vi "get results and parameters refs.vi"(8 "error in":errorcluster, 11 "VI in":refnum<vi>) -> (0 "error out":errorcluster, 2 "Results from processing ref out":refnum<vi>, 3 "Parameters to process ref out":refnum<vi>)   [LabVIEW 2013]
uses:
  <vilib>/Utility/traverseref.llb/TRef TravTarget.ctl
  <vilib>/Utility/traverseref.llb/VI Scripting - Traverse.lvlib
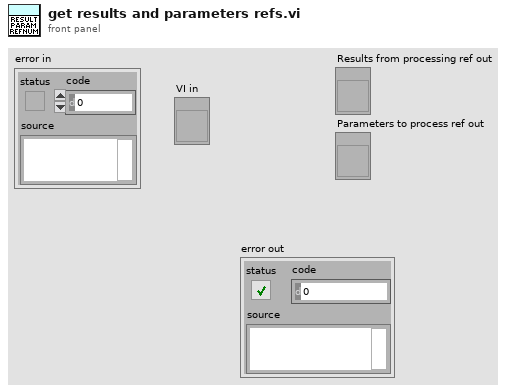
[diagram p1: front panel]
types:
  T1 = typedef "TRef TravTarget.ctl" = enum16{"FP", "BD", "Other"}
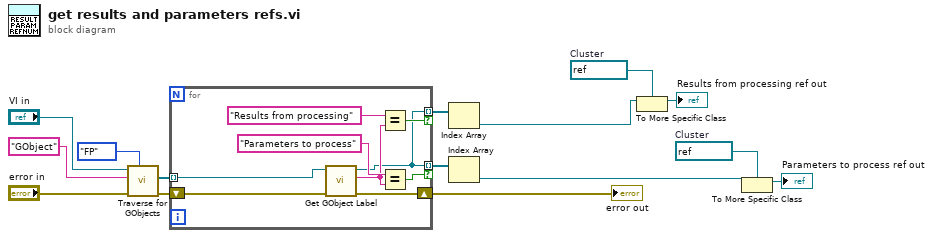
[diagram p0: block diagram]
diagram:
  w4 = refnum<vi> refnum  # Cluster
  w5 = refnum<vi> refnum  # Cluster
  n1 = call <vilib>:"Traverse for GObjects.vi"("Traverse Target"=TRef_TravTarget."FP", "error in (no error)"="error in", "Class Name"="GObject", "VI Refnum"="VI in") -> ("error out"=w14:errorcluster, "References"=w10:refnum<vi>[])  [unwired: 4 in, 2 out]
  n2 = for {
    tunnel: [w18] -> w12 mode=indexing if=w22
    shift-right: [w21] -> w13
    shift-left: w14 -> [w24]
    tunnel: [w18] -> w11 mode=indexing if=w17
    tunnel: w10 -> [w16] mode=indexing
    n3 = call <vilib>:"Get GObject Label.vi"("error in (no error)"=w24, "GObject"=w16) -> ("error out"=w21:errorcluster, "Object Label"=w19:string, "dup GObject"=w18:refnum<vi>)  [unwired: 5 in, 2 out]
    n4 = Equal?(x="Results from processing", y=w19) -> (x = y?=w22:bool)
    n5 = Equal?(x="Parameters to process", y=w19) -> (x = y?=w17:bool)
  }
  "error out" <- w13
  n6 = Index Array(array=w12) -> (element=w6:refnum<vi>)  [unwired: 1 in]
  n7 = Index Array(array=w11) -> (element=w3:refnum<vi>)  [unwired: 1 in]
  n8 = To More Specific Class(target class=w5, reference=w6) -> (specific class reference=→"Results from processing ref out":refnum<vi>)  [unwired: 1 in, 1 out]
  n9 = To More Specific Class(target class=w4, reference=w3) -> (specific class reference=→"Parameters to process ref out":refnum<vi>)  [unwired: 1 in, 1 out]
